vi "Get Shell Speed.vi"(0 "loading":sgl format="%.2f", 1 "v50":sgl=450.0 format="%.2f") -> (3 "impact":sgl=1591.9158 format="%.2f", 4 "residual":sgl=795.9579 format="%.2f", 5 "SECONDS":sgl=3246548700.0)   [LabVIEW 2015]
panel:
  in  "scale":sgl=3.0 format="%.2f"
  out "velocity":sgl(graph)=1591.9158
  in  "y":sgl=0.5
  # "Private"
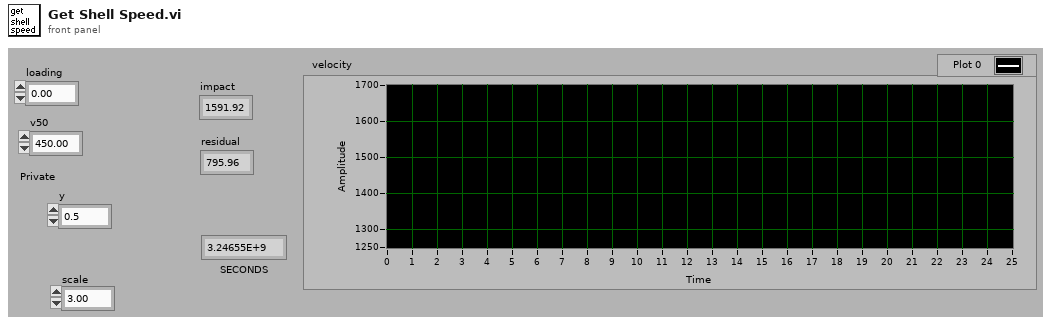
[diagram p1: front panel]
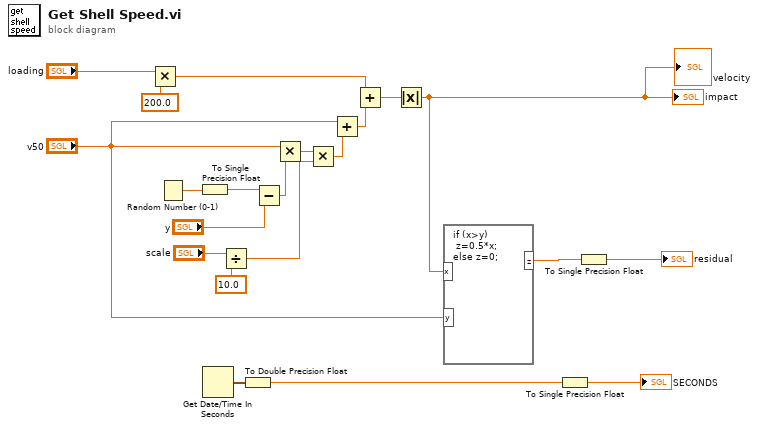
[diagram p0: block diagram]
diagram:
  n1 = Multiply(x="loading", y=sgl 200.0) -> (x*y=w18:sgl)
  n2 = Random Number (0-1)() -> (number: 0 to 1=w16:dbl)
  n3 = To Single Precision Float(number=w16) -> (single precision float=w10:sgl)
  n4 = Get Date/Time In Seconds() -> (seconds since 1Jan1904=w11:timestamp)
  n5 = Divide(x="scale", y=sgl 10.0) -> (x/y=w4:sgl)
  n6 = To Double Precision Float(number=w11) -> (double precision float=w14:dbl)
  n7 = Subtract(x=w10, y="y") -> (x-y=w15:sgl)
  n8 = Multiply(x="v50", y=w15) -> (x*y=w21:sgl)
  n9 = Multiply(x=w21, y=w4) -> (x*y=w2:sgl)
  n10 = Add(x="v50", y=w2) -> (x+y=w3:sgl)
  n11 = Add(x=w18, y=w3) -> (x+y=w12:sgl)
  n12 = Absolute Value(x=w12) -> (abs(x)=w7:sgl)
  "impact" <- w7
  "velocity" <- w7
  n13 = formula code="if (x>y)\n z=0.5*x;\nelse z=0;"("x"=w7, "y"="v50") -> ("z"=w13:dbl)
  n14 = To Single Precision Float(number=w14) -> (single precision float=→"SECONDS":sgl)
  n15 = To Single Precision Float(number=w13) -> (single precision float=→"residual":sgl)
